vi "Float32 Get Byte.vi"(8 "error in (no error)":errorcluster, 11 "Float32 DVR in":refnum<data-value>) -> (0 "error out":errorcluster, 2 "I8 out":i8, 3 "Float32 DVR out":refnum<data-value>)   [LabVIEW 2010, in "MDSplus.lvlib"]
uses:
  <vilib>/MDSplus/Library/MDSplus.lvlib
  <vilib>/MDSplus/Classes/Data_Class/Scalar_Class/Float32_Class/Float32.lvclass
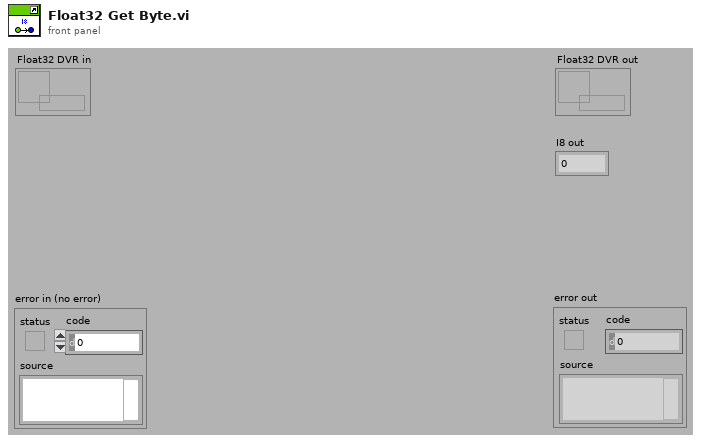
[diagram p1: front panel]
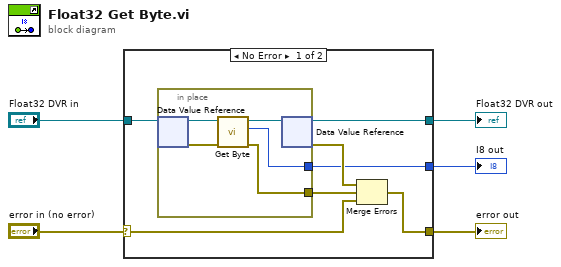
[diagram p0: block diagram]
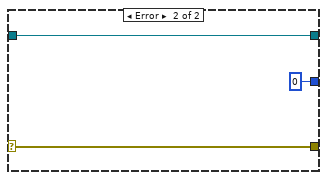
[diagram p2: hidden frame]
diagram:
  n1 = case shown="No Error" "error in (no error)" {
    selector: "error in (no error)" -> [w10 w19]
    tunnel: "Float32 DVR in" -> [w12 w18]
    tunnel: [w8 w19] -> w5
    tunnel: [w7 w18] -> w1
    tunnel: [w6 i8 0 ("Float out")] -> w4
    frame No Error {
      n2 = in-place {
        in-place-border: [w15] -> w11
        in-place-border: [w13] -> w6
        n3 = in-place-dvr #1(w12) -> (w17:refnum<class "Float32.lvclass">, w14:errorcluster)
        n4 = call-dynamic "Get Byte.vi"("error in (no error)"=w14, "Float32 in"=w17) -> ("error out"=w15:errorcluster, "I8 out"=w13:i8, "Float32 out"=w16:refnum<class "Float32.lvclass">)  [unwired: 7 in]
        n5 = in-place-dvr #1(w16) -> (w7:refnum<data-value>, w9:errorcluster)
      }
      n6 = Merge Errors(w9, w11, w10) -> (w8:errorcluster)
    }
    frame Error {
    }
  }
  "error out" <- w5
  "I8 out" <- w4
  "Float32 DVR out" <- w1
